vi "Shift Input.vi"(7 "Control":refnum<vi>, 8 "Error In":errorcluster, 9 "Panel Height":i32, 10 "Panel Width":i32, 11 "Pop Up ref":refnum<vi>) -> (0 "Error Out":errorcluster, 1 "Panel Height out":i32, 2 "Panel Width out":i32)   [LabVIEW 2021, in "Pop-Up.lvlib" / "Popup.lvclass"]
doc: "move the input down to the correct position and shift the front panel size and location for input button if needed\n\n<b>Code Developed By:</b> +\nDaniel Coons +\nhttps://github.com/danielcoons/tsc-pop-up"
uses:
  Popup.lvclass
  <vilib>/Utility/miscctls.llb/LVPositionTypeDef.ctl
  Popup.lvclass/Popup.ctl
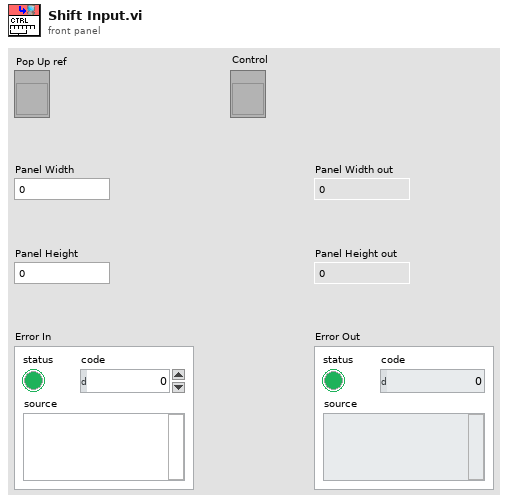
[diagram p1: front panel]
types:
  T1 = typedef "LVRectTypeDef.ctl" = cluster{"Left":i16, "Top":i16, "Right":i16, "Bottom":i16}
  T2 = typedef "LVPositionTypeDef.ctl" = cluster{"Left":i32, "Top":i32}
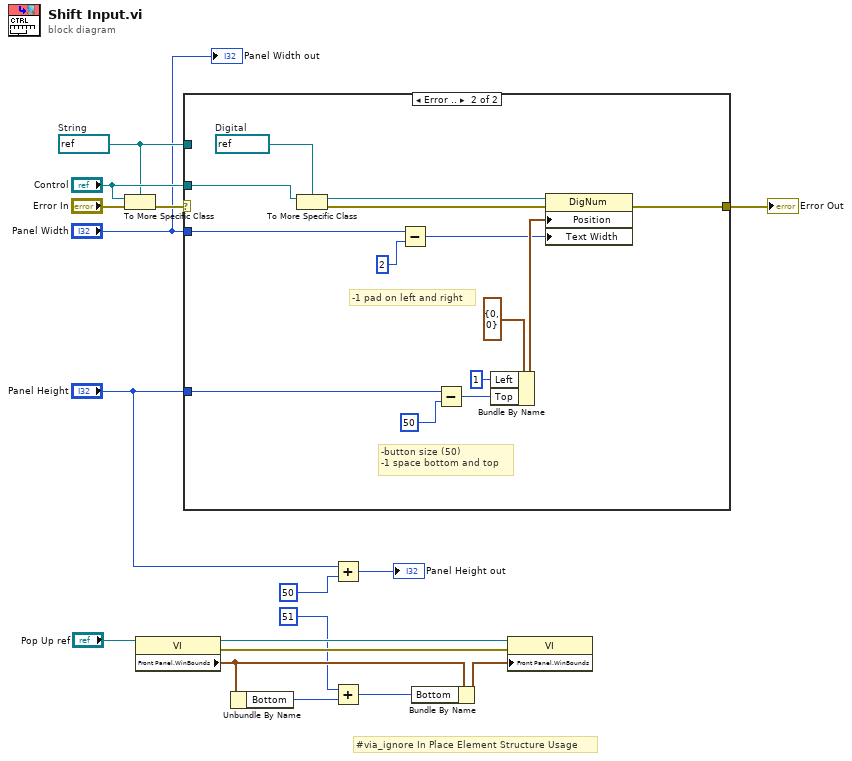
[diagram p0: block diagram]
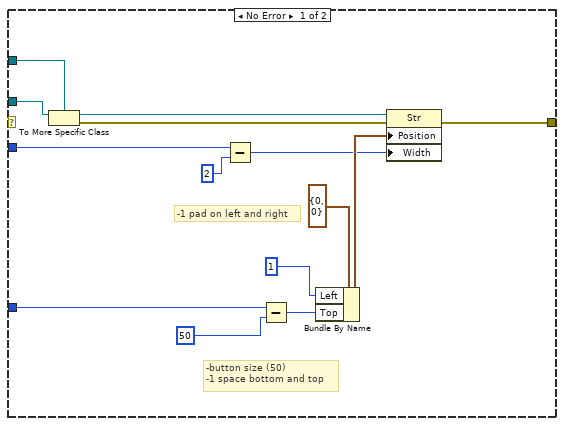
[diagram p2: hidden frame]
diagram:
  w13 = refnum<vi> refnum  # String
  # "#via_ignore In Place Element Structure Usage"
  n1 = To More Specific Class(target class=w13, reference="Control", error in="Error In") -> (error out=w15:errorcluster)  [unwired: 1 out]
  n2 = property class="VI"(reference="Pop Up ref") -> (reference out=w6:refnum<vi>, error out=w7:errorcluster, "Front Panel.WinBounds"=w8:T1)  [unwired: 1 in]
  n3 = case shown="Error .." w15 {
    tunnel: [w30 w44] -> w17
    tunnel: "Panel Height" -> [w29 w43]
    tunnel: "Panel Width" -> [w24 w38]
    tunnel: "Control" -> [w21 w35]
    tunnel: w13 -> [w20 _]
    frame No Error {
      # "-button size (50)\n-1 space bottom and top"
      # "-1 pad on left and right"
      n4 = To More Specific Class(target class=w20, reference=w21) -> (specific class reference=w19:refnum<vi>, error out=w18:errorcluster)  [unwired: 1 in]
      n5 = Subtract(x=w24, y=2) -> (x-y=w23:i32)
      n6 = Subtract(x=w29, y=50) -> (x-y=w25:i32)
      n7 = Bundle By Name(cluster=T2 {"Left"=0, "Top"=0} ("Position"), "Left"=1, "Top"=w25) -> (w26:T2)
      n8 = property class="Str"(reference=w19, error in=w18, "Position"=w26, "Width"=w23) -> (error out=w30:errorcluster)  [unwired: 1 out]
    }
    frame Error {
      w32 = refnum<vi> refnum  # Digital
      # "-button size (50)\n-1 space bottom and top"
      # "-1 pad on left and right"
      n9 = To More Specific Class(target class=w32, reference=w35) -> (specific class reference=w34:refnum<vi>, error out=w33:errorcluster)  [unwired: 1 in]
      n10 = Subtract(x=w38, y=2) -> (x-y=w37:i32)
      n11 = Subtract(x=w43, y=50) -> (x-y=w39:i32)
      n12 = Bundle By Name(cluster=T2 {"Left"=0, "Top"=0} ("Position"), "Left"=1, "Top"=w39) -> (w40:T2)
      n13 = property class="DigNum"(reference=w34, error in=w33, "Position"=w40, "Text Width"=w37) -> (error out=w44:errorcluster)  [unwired: 1 out]
    }
  }
  "Error Out" <- w17
  n14 = Unbundle By Name(w8) -> ("Bottom"=w4:i16)
  n15 = Add(x="Panel Height", y=50) -> (x+y=→"Panel Height out":i32)
  n16 = Add(x=51 ("y"), y=w4) -> (x+y=w3:i32)
  n17 = Bundle By Name(cluster=w8, "Bottom"=w3) -> (w5:T1)
  n18 = property class="VI"(reference=w6, error in=w7, "Front Panel.WinBounds"=w5) -> ()  [unwired: 2 out]
  "Panel Width out" <- "Panel Width"
